vi "SaveLineout.vi"(11 "Refnum in":T1) -> (2 "Y Axis Averages":sgl[](array[numeric]) format="%.2f", 3 "X Axis Averages":sgl[](array[numeric]) format="%.2f")   [LabVIEW 2011, in "MoveDataFile.lvclass"]
uses:
  MoveDataFile.lvclass
  <vilib>/vision/Image Controls.llb/IMAQ Image.ctl
  shared/CompressAndUpdate(Poly)/CompressAndUpdate(NumericArray).vi
  <vilib>/vision/NI_Vision_Development_Module.lvlib
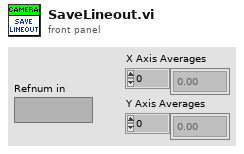
[diagram p1: front panel]
types:
  T1 = typedef "IMAQ Image.ctl" = refnum<image>
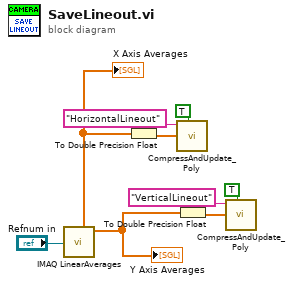
[diagram p0: block diagram]
diagram:
  n1 = call "IMAQ LinearAverages"("Image Src"="Refnum in") -> ("Y Axis Averages"=w5:sgl[], "X Axis Averages"=w9:sgl[])  [unwired: 6 in, 3 out]
  "X Axis Averages" <- w9
  "Y Axis Averages" <- w5
  n2 = To Double Precision Float(number=w9) -> (double precision float=w6:dbl[])
  n3 = call-poly "CompressAndUpdate_Poly.vi"("force CVT update (false)"=TRUE ("force CVT update"), "Numeric Array"=w6, "command or variable name"="HorizontalLineout") -> ()  [unwired: 8 in, 1 out]
  n4 = To Double Precision Float(number=w5) -> (double precision float=w4:dbl[])
  n5 = call-poly "CompressAndUpdate_Poly.vi"("force CVT update (false)"=TRUE ("force CVT update"), "Numeric Array"=w4, "command or variable name"="VerticalLineout") -> ()  [unwired: 8 in, 1 out]
